vi "Subsystem Sequencer Controller.vi"(8 "error in":errorcluster) -> ()   [LabVIEW 2019]
doc: "This VI executes continuously carrying out the current operation and responding to updates or new operations. It will often contain the timing or control code that is difficult to place directly in TeleOp. This VI generally opens all sensors and motors and isolates the rest of the robot code from knowing how the operations are carried out."
uses:
  <vilib>/Rock Robotics/WPI/Framework/Completion Status.ctl
  Subsystem Sequencer Setpoints.ctl
  Subsystem Sequencer Operations.ctl
  All Commands.ctl
  <vilib>/Rock Robotics/SystemInterfaces/AI/FPGA_AIChannel.ctl
  Sequencer Type.ctl
panel:
  in  "Shoot Position":dbl=31.0 format="%#_13g"
  in  "Pickup Position":dbl format="%#_13g"
  out "Value":dbl
  out "Cmd":T1
  out "Waveform Chart":T2(graph)
  in  "Sensor Cube Threshold":dbl=1.55 format="%#_13g"
  in  "Interactive Values":T3
  out "Current\nCmd":string
  in  "Buttons":cluster{"Execute Cmd":bool, "Abort Cmd":bool}
  out "Command Timing":cluster{"Start Time (ms)":u32, "Iterations":i32}
  out "Status":T5
  # "Interactive Command: You may fill in the settings for a command\nand schedule it with the Execute button. You can observe and abort\nany command while fine tuning the code for the controller."
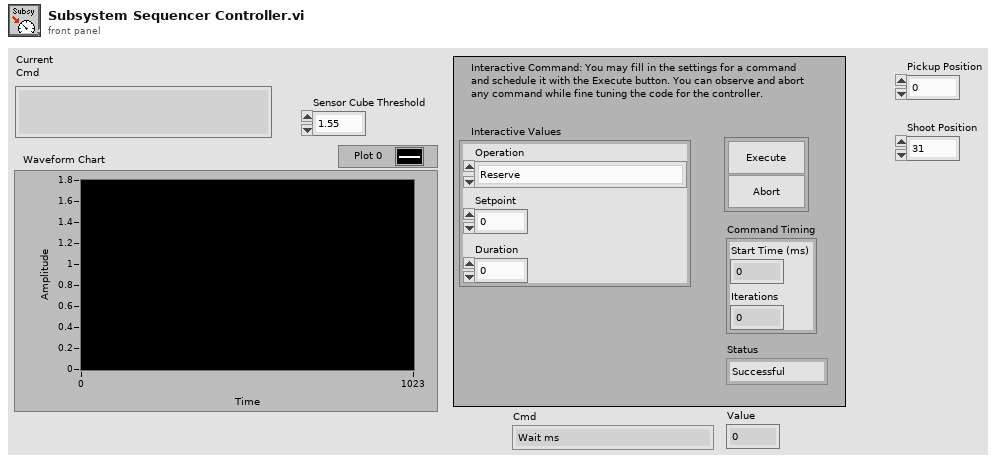
[diagram p1: front panel]
types:
  T1 = typedef "All Commands.ctl" = enum16{"Wait ms", "Drive - Stop Driving", "Drive - Set Shifter", "Drive - Drive Distance Straight", "Elevator - Elevator Stop", "Elevator - Elevator Set Position Wait", "Elevator - Elevator Set Position Start", "Arm - Arm to Shoot Position", "Arm - Arm to Pickup Position", "Arm - Arm Set Position", "Gripper - Gripper Stop", "Gripper - Gripper Shoot", "Gripper - Gripper Open", "Gripper - Gripper Intake", "Gripper - Gripper Close", "Gripper - Wait on Sensor"}
  T2 = cluster{"Sensor Cube Threshold":dbl, "Voltage":dbl}
  T3 = typedef "Subsystem Sequencer Setpoints.ctl" = cluster{"Operation":T4, "Setpoint":dbl, "Duration":dbl}
  T4 = typedef "Subsystem Sequencer Operations.ctl" = enum16{"Reserve", "Read Current", "Run Sequence"}
  T5 = typedef "Completion Status.ctl" = enum16{"Successful", "Aborted", "Incomplete"}
  T6 = typedef "FPGA_AIChannel.ctl" = enum8{"AI 0", "AI 1", "AI 2", "AI 3", "AI MXP 0", "AI MXP 1", "AI MXP 2", "AI MXP 3", "Invalid"}
  T7 = typedef "WPI_AnalogChannelDevRef.ctl" = cluster{"DevStatus":errorcluster, "Analog Channel":T6}
  T8 = typedef "Command Status Info.ctl" = cluster{"Name":string, "Status":T5, "notifier out":T9}
  T9 = typedef "Completion Notifier.ctl" = refnum<notifier>
  T10 = cluster{"Current Command":T3, "Command Timing":cluster{"Start Time (ms)":u32, "Iterations":i32}, "Command Arguments":cluster{"Command Info":T8, "Description":string, "Default Command":T3, "queue out":refnum<queue>, "Subsystem Name":string}}
  T11 = typedef "Sequencer Type.ctl" = cluster{"Cmd":T1, "Value":dbl}
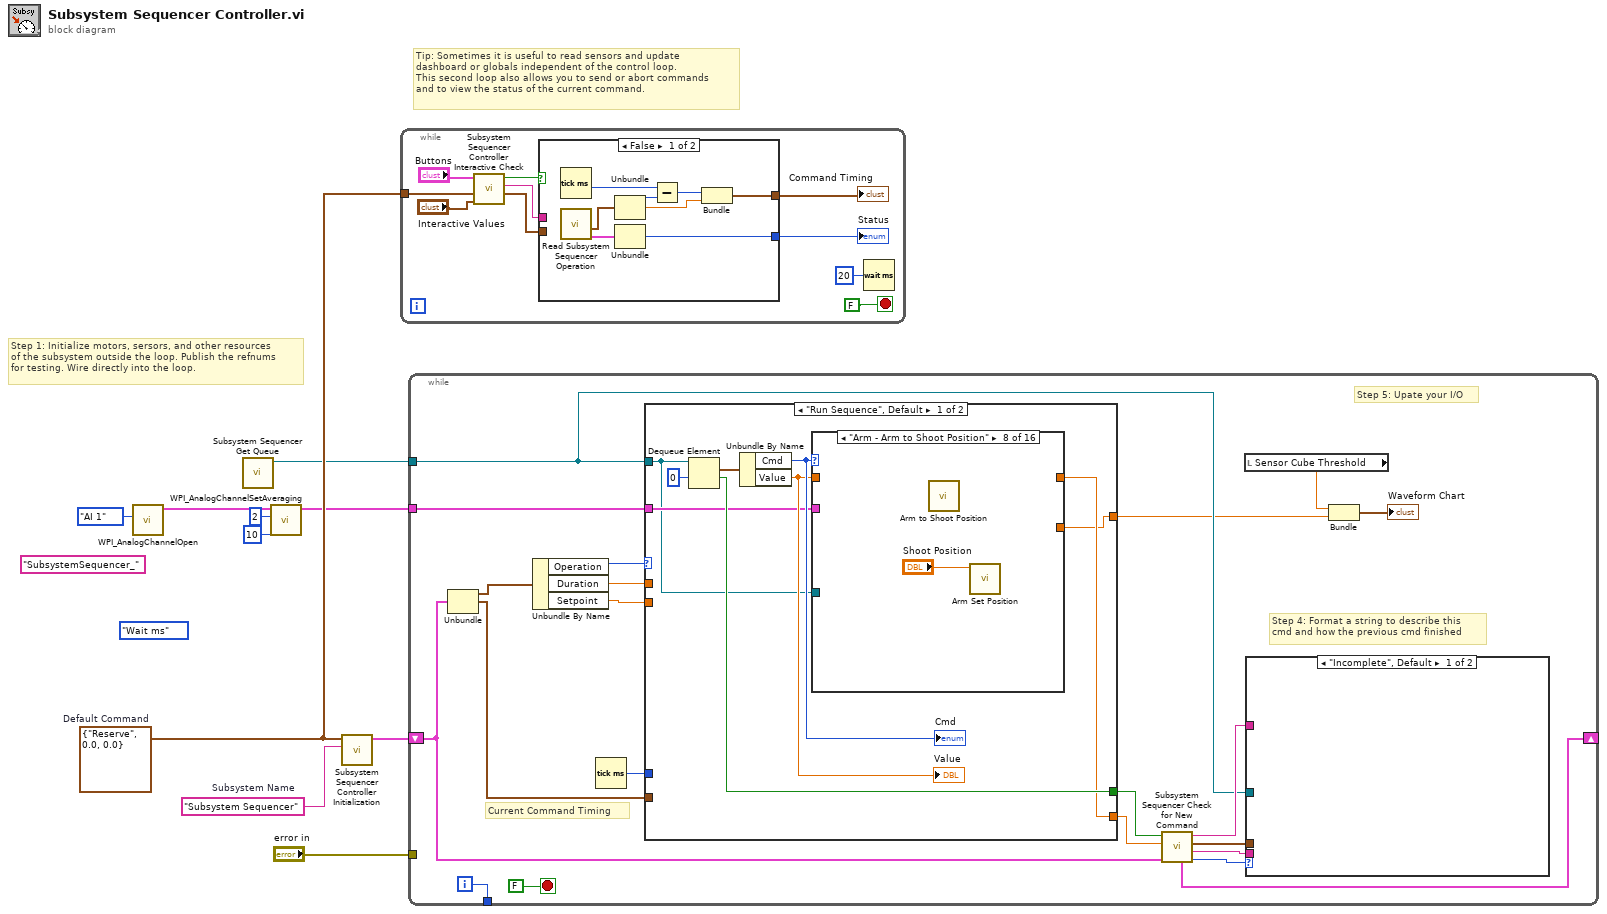
[diagram p0: block diagram]
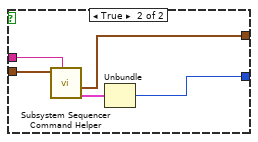
[diagram p2: hidden frame]
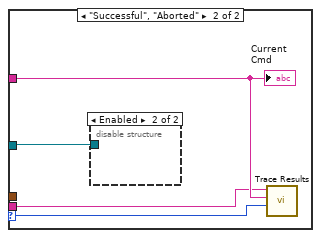
[diagram p3: hidden frame]
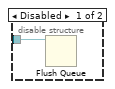
[diagram p4: hidden frame]
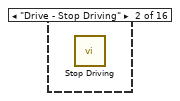
[diagram p6: hidden frame]
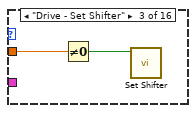
[diagram p7: hidden frame]
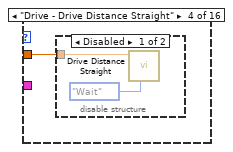
[diagram p8: hidden frame]
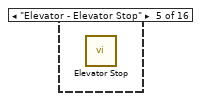
[diagram p10: hidden frame]
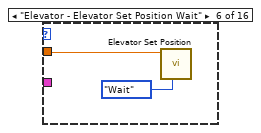
[diagram p11: hidden frame]
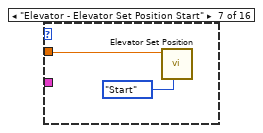
[diagram p12: hidden frame]
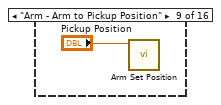
[diagram p13: hidden frame]
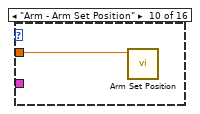
[diagram p14: hidden frame]
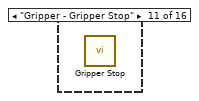
[diagram p15: hidden frame]
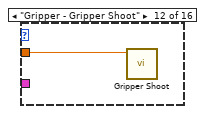
[diagram p16: hidden frame]
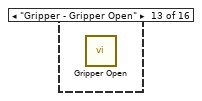
[diagram p17: hidden frame]
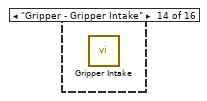
[diagram p18: hidden frame]
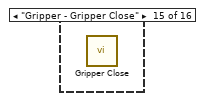
[diagram p19: hidden frame]
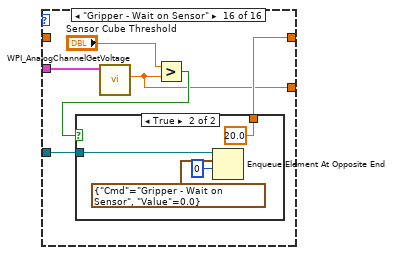
[diagram p20: hidden frame]
diagram:
  (unwired) "SubsystemSequencer_" ("name (unnamed)")
  (unwired) All_Commands."Wait ms" ("Cmd")
  w7 = T3 {"Operation"=enum."Reserve", "Setpoint"=0.0, "Duration"=0.0}  # Default Command
  w8 = "Subsystem Sequencer"  # Subsystem Name
  # "Tip: Sometimes it is useful to read sensors and update\ndashboard or globals independent of the control loop.\nThis second loop also allows you to send or abort commands\nand to view the status of the current command."
  # "Step 1: Initialize motors, sersors, and other resources\nof the subsystem outside the loop. Publish the refnums\nfor testing. Wire directly into the loop."
  n1 = call <vilib>:"WPI_AnalogChannelOpen.vi"("Analog Channel"=FPGA_AIChannel."AI 1") -> ("AIDeviceRef"=w5:T7)  [unwired: 9 in, 1 out]
  n2 = call "Subsystem Sequencer Get Queue.vi"() -> ("queue out"=w4:refnum<queue>)  [unwired: 10 in, 1 out]
  n3 = call <vilib>:"WPI_AnalogChannelSetAveraging.vi"("OversampleBits"=u8 10, "AverageBits"=u8 2, "AIDeviceRef"=w5) -> ("AIDeviceRef"=w3:T7)  [unwired: 7 in, 1 out]
  n4 = call "Subsystem Sequencer Controller Initialization.vi"("Subsystem Name"=w8, "Default Command"=w7) -> ("Current Command"=w9:T10)  [unwired: 9 in]
  n5 = while {
    tunnel: w7 -> [w17]
    stop <- FALSE stop-if-true
    n6 = call "Subsystem Sequencer Controller Interactive Check.vi"("Interactive Command in"="Interactive Values", "Default Command"=w17, "Buttons"="Buttons") -> ("Interactive Command out"=w14:T3, "Trace String"=w15:string, "Schedule"=w16:bool)  [unwired: 6 in]
    n7 = case shown="False" w16 {
      tunnel: [w28 w33] -> w13
      tunnel: w14 -> [_ w31]
      tunnel: [w24 w29] -> w12
      tunnel: w15 -> [_ w32]
      frame False {
        n8 = Tick Count (ms)() -> (millisecond timer value=w23:u32)
        n9 = call "Read Subsystem Sequencer Operation.vi"() -> ("Command Info"=w21:T8, "SubSystem Data"=w22:T3)  [unwired: 9 in, 1 out]
        n10 = Unbundle(w22) -> ("Operation"=w27:T4, "Setpoint"=w25:dbl)  [unwired: 1 out]
        n11 = Unbundle(w21) -> ("Status"=w28:T5)  [unwired: 2 out]
        n12 = Subtract(x=w23, y=w27) -> (x-y=w26:u32)
        n13 = Bundle(w26, "Setpoint"=w25) -> (w24:cluster{u32, "Setpoint":dbl})  [unwired: 1 in]
      }
      frame True {
        n14 = call "Subsystem Sequencer Command Helper.vi"("Description"=w32, "SubSystem Data"=w31) -> ("Command Info Out"=w30:T8, "Command Timing"=w29:cluster{"Start Time (ms)":u32, "Iterations":i32})  [unwired: 7 in, 1 out]
        n15 = Unbundle(w30) -> ("Status"=w33:T5)  [unwired: 2 out]
      }
    }
    "Status" <- w13
    "Command Timing" <- w12
    n16 = Wait (ms)(milliseconds to wait=u32 20) -> ()  [unwired: 1 out]
  }
  n17 = while {
    shift-right: [w46] -> _
    shift-left: w9 -> [w39]
    tunnel: [w53] -> _
    tunnel: "error in" -> [_]
    tunnel: w4 -> [w38]
    tunnel: w3 -> [w37]
    i -> [w53]
    stop <- FALSE stop-if-true
    # "Step 5: Upate your I/O"
    # "Step 4: Format a string to describe this\ncmd and how the previous cmd finished"
    # "Current Command Timing"
    n18 = Unbundle(w39) -> ("Current Command"=w52:T3, "Command Timing"=w48:cluster{"Start Time (ms)":u32, "Iterations":i32})  [unwired: 1 out]
    n19 = Unbundle By Name(w52) -> ("Operation"=w51:T4, "Duration"=w50:dbl, "Setpoint"=w47:dbl)
    n20 = Tick Count (ms)() -> (millisecond timer value=w49:u32)
    n21 = case shown="\"Run Sequence\", Default" w51 {
      tunnel: [w63 w96] -> w44
      tunnel: [w67 FALSE ("ignore previous (F)")] -> w45
      tunnel: w48 -> [_ _]
      tunnel: w50 -> [_ _]
      tunnel: w49 -> [_ _]
      tunnel: w47 -> [_ _]
      tunnel: w38 -> [w61 _]
      tunnel: w37 -> [w62 w94]
      tunnel: [w60 w93] -> w36
      frame "Run Sequence", Default {
        n22 = Dequeue Element(queue=w61, timeout in ms (-1)=0) -> (element=w66:T11, timed out?=w67:bool)  [unwired: 1 in, 2 out]
        n23 = Unbundle By Name(w66) -> ("Cmd"=w65:T1, "Value"=w64:dbl)
        "Cmd" <- w65
        "Value" <- w64
        n24 = case shown="\"Arm - Arm to Shoot Position\"" w65 {
          tunnel: w64 -> [w69 _ w71 w72 _ w76 w78 _ _ w81 _ w82 _ _ _ _]
          tunnel: [w69 _ _ _ _ _ _ _ _ _ _ _ _ _ _ w84] -> w63
          tunnel: w62 -> [_ _ _ _ _ _ _ _ _ _ _ _ _ _ _ w88]
          tunnel: w61 -> [_ _ _ _ _ _ _ _ _ _ _ _ _ _ _ w86]
          tunnel: [_ _ _ _ _ _ _ _ _ _ _ _ _ _ _ w83] -> w60
          frame "Wait ms", Default {
          }
          frame "Drive - Stop Driving" {
            n25 = call "Stop Driving.vi"() -> ()  [unwired: 11 in, 1 out]
          }
          frame "Drive - Set Shifter" {
            n26 = Not Equal To 0?(x=w71) -> (x != 0?=w70:bool)
            n27 = call "Set Shifter.vi"("High Gear?"=w70) -> ()  [unwired: 10 in, 1 out]
          }
          frame "Drive - Drive Distance Straight" {
            n28 = disable-structure shown="Disabled" {
              disable-tunnel: w72 -> [w74 _]
              frame Disabled {
                n29 = call "Drive Distance Straight.vi"("Synchronication"=enum16{"Start", "Wait"}."Wait", "Distance"=w74) -> ()  [unwired: 9 in, 1 out]
              }
              frame Enabled {
              }
            }
          }
          frame "Elevator - Elevator Stop" {
            n30 = call "Elevator Stop.vi"() -> ()  [unwired: 11 in, 1 out]
          }
          frame "Elevator - Elevator Set Position Wait" {
            n31 = call "Elevator Set Position.vi"("Synchronization"=enum16{"Start", "Wait"}."Wait", "Setpoint"=w76) -> ()  [unwired: 9 in, 1 out]
          }
          frame "Elevator - Elevator Set Position Start" {
            n32 = call "Elevator Set Position.vi"("Synchronization"=enum16{"Start", "Wait"}."Start", "Setpoint"=w78) -> ()  [unwired: 9 in, 1 out]
          }
          frame "Arm - Arm to Shoot Position" {
            n33 = call "Arm to Shoot Position.vi"() -> ()  [unwired: 11 in, 1 out]
            n34 = call "Arm Set Position.vi"("Setpoint"="Shoot Position") -> ()  [unwired: 10 in, 1 out]
          }
          frame "Arm - Arm to Pickup Position" {
            n35 = call "Arm Set Position.vi"("Setpoint"="Pickup Position") -> ()  [unwired: 10 in, 1 out]
          }
          frame "Arm - Arm Set Position" {
            n36 = call "Arm Set Position.vi"("Setpoint"=w81) -> ()  [unwired: 10 in, 1 out]
          }
          frame "Gripper - Gripper Stop" {
            n37 = call "Gripper Stop.vi"() -> ()  [unwired: 11 in, 1 out]
          }
          frame "Gripper - Gripper Shoot" {
            n38 = call "Gripper Shoot.vi"("Speed (1)"=w82) -> ()  [unwired: 10 in, 1 out]
          }
          frame "Gripper - Gripper Open" {
            n39 = call "Gripper Open.vi"() -> ()  [unwired: 11 in, 1 out]
          }
          frame "Gripper - Gripper Intake" {
            n40 = call "Gripper Intake.vi"() -> ()  [unwired: 11 in, 1 out]
          }
          frame "Gripper - Gripper Close" {
            n41 = call "Gripper Close.vi"() -> ()  [unwired: 11 in, 1 out]
          }
          frame "Gripper - Wait on Sensor" {
            n42 = call <vilib>:"WPI_AnalogChannelGetVoltage.vi"("AIDeviceRef"=w88) -> ("Voltage"=w83:dbl)  [unwired: 8 in, 2 out]
            n43 = Greater?(x="Sensor Cube Threshold", y=w83) -> (0:w85:bool)
            n44 = case shown="True" w85 {
              tunnel: w86 -> [_ w92]
              tunnel: [_ 20.0 ("Value")] -> w84
              frame False {
              }
              frame True {
                n45 = Enqueue Element At Opposite End(queue=w92, element=T11 {"Cmd"=enum."Gripper - Wait on Sensor", "Value"=0.0}, timeout in ms (-1)=0) -> ()  [unwired: 1 in, 3 out]
              }
            }
          }
        }
      }
      frame "Reserve" {
        w96 = 100.0  # Infinite
        # "For debugging the sensor"
        n46 = call <vilib>:"WPI_AnalogChannelGetVoltage.vi"("AIDeviceRef"=w94) -> ("Voltage"=w93:dbl)  [unwired: 8 in, 2 out]
      }
    }
    n47 = call "Subsystem Sequencer Check for New Command.vi"("Current Command"=w39, "Wait time (ms)"=w44, "Finished?"=w45) -> ("Completion"=w40:T5, "Subsystem Name"=w41:string, "Current Command"=w42:T3, "Initial Trace String"=w43:string, "NextCommand"=w46:T10)  [unwired: 4 in]
    n48 = local read "Sensor Cube Threshold"() -> (w34:dbl)
    n49 = case shown="\"Incomplete\", Default" w40 {
      selector: w40 -> [_ w58]
      tunnel: w43 -> [_ w57]
      tunnel: w42 -> [_ _]
      tunnel: w41 -> [_ w56]
      tunnel: w38 -> [_ w55]
      frame "Incomplete", Default {
        # "Continuing current command"
      }
      frame "Successful", "Aborted" {
        # "Report and setup for next command"
        n50 = disable-structure shown="Enabled" {
          disable-tunnel: w55 -> [w59 _]
          frame Disabled {
            n51 = Flush Queue(queue=w59) -> ()  [unwired: 1 in, 3 out]
          }
          frame Enabled {
          }
        }
        n52 = call <vilib>:"Trace Results.vi"("Status of previous command"=w58, "Description"=w57, "Subsystem"=w56) -> ()  [unwired: 9 in]
        "Current\nCmd" <- w57
      }
    }
    n53 = Bundle("Sensor Cube Threshold"=w34, "Voltage"=w36) -> (→"Waveform Chart":T2)  [unwired: 1 in]
  }
